vi "practiceImageAnalysis.vi"() -> ()   [LabVIEW 2016]
uses:
  <vilib>/regexp/Match Regular Expression.xnode
  <vilib>/Utility/file.llb/Write Delimited Spreadsheet (DBL).vi
  <vilib>/vision/Measure.llb/Straight Edge Process.ctl
  <vilib>/vision/Measure.llb/Straight Edge Options.ctl
  <vilib>/vision/Measure.llb/Edge Polarity.ctl
  <vilib>/vision/Measure.llb/Edge Options.ctl
panel:
  out "Coordinate array for image capture":dbl[][](array[numeric])
  in  "Coordinate file for image capture":path=path "E:/XYZstage+Camera_CollectedImages/12-16-2016/noStaveMount/toolingpinsCoordinates-captured.csv"
  out "Review":bool
  out "Search running?":bool
  in  "Options: Bottom Edge Search":T3={"Search Direction"=3, "Edge Options"={"Edge Polarity"=2, "Kernel Size"=9, "Width"=3, "Minimum Edge Strength"=17.0, "Interpolation Type"=enum."Bilinear Fixed", "Data Processing Method"=enum."Average"}, "Show Search Area"=TRUE, "Show Search Lines"=TRUE, "Show Edges Found"=TRUE, "Show Result"=TRUE, "Search Area Color"=65280, "Search Lines Color"=255, "Edge Locations Color"=16776960, "Result Color"=16711680, "Overlay Group Name"=""} {"Search Direction" items=["Left to Right", "Right to Left", "Top to Bottom", "Bottom to Top"]; "Edge Options"."Edge Polarity" items=["All Edges", "Rising Edges", "Falling Edges"]; "Edge Options"."Minimum Edge Strength" format="%.2f"; "Edge Options"."Width" step=2; "Edge Options"."Kernel Size" step=2}
  in  "Options: Top Edge Search":T3={"Search Direction"=2, "Edge Options"={"Edge Polarity"=0, "Kernel Size"=5, "Width"=3, "Minimum Edge Strength"=16.0, "Interpolation Type"=enum."Bilinear Fixed", "Data Processing Method"=enum."Average"}, "Show Search Area"=TRUE, "Show Search Lines"=TRUE, "Show Edges Found"=TRUE, "Show Result"=TRUE, "Search Area Color"=65280, "Search Lines Color"=255, "Edge Locations Color"=16776960, "Result Color"=16711680, "Overlay Group Name"=""} {"Search Direction" items=["Left to Right", "Right to Left", "Top to Bottom", "Bottom to Top"]; "Edge Options"."Edge Polarity" items=["All Edges", "Rising Edges", "Falling Edges"]; "Edge Options"."Minimum Edge Strength" format="%.2f"; "Edge Options"."Width" step=2; "Edge Options"."Kernel Size" step=2}
  in  "Fit Options":T4={"Number of Lines"=1, "Type"=enum."First Edge Rake", "Min. Score"=10.0, "Max. Score"=1000.0, "Orientation"=0.0, "Angle Range"=45.0, "Angle Tolerance"=1.0, "Step Size"=196, "Min. SNR (db)"=0.0, "Min. Points (%)"=25.0, "Hough Iterations"=5} {"Min. Points (%)" min=0.0 max=100.0; "Min. SNR (db)" min=0.0; "Max. Score" min=0.0 max=1024.0; "Min. Score" min=0.0 max=1024.0 step=1.0}
  in  "Stop and delete":bool
  out "Images Array":T6[](array[plugin-control])
  in  "error in":errorcluster
  out "error out":errorcluster
  out "Filenames Array":string[](array[string])
  in  "Naming Convention":string="*.png"
  in  "Images Directory":path=path "E:/XYZstage+Camera_CollectedImages/12-16-2016/noStaveMount/toolingpins_images"
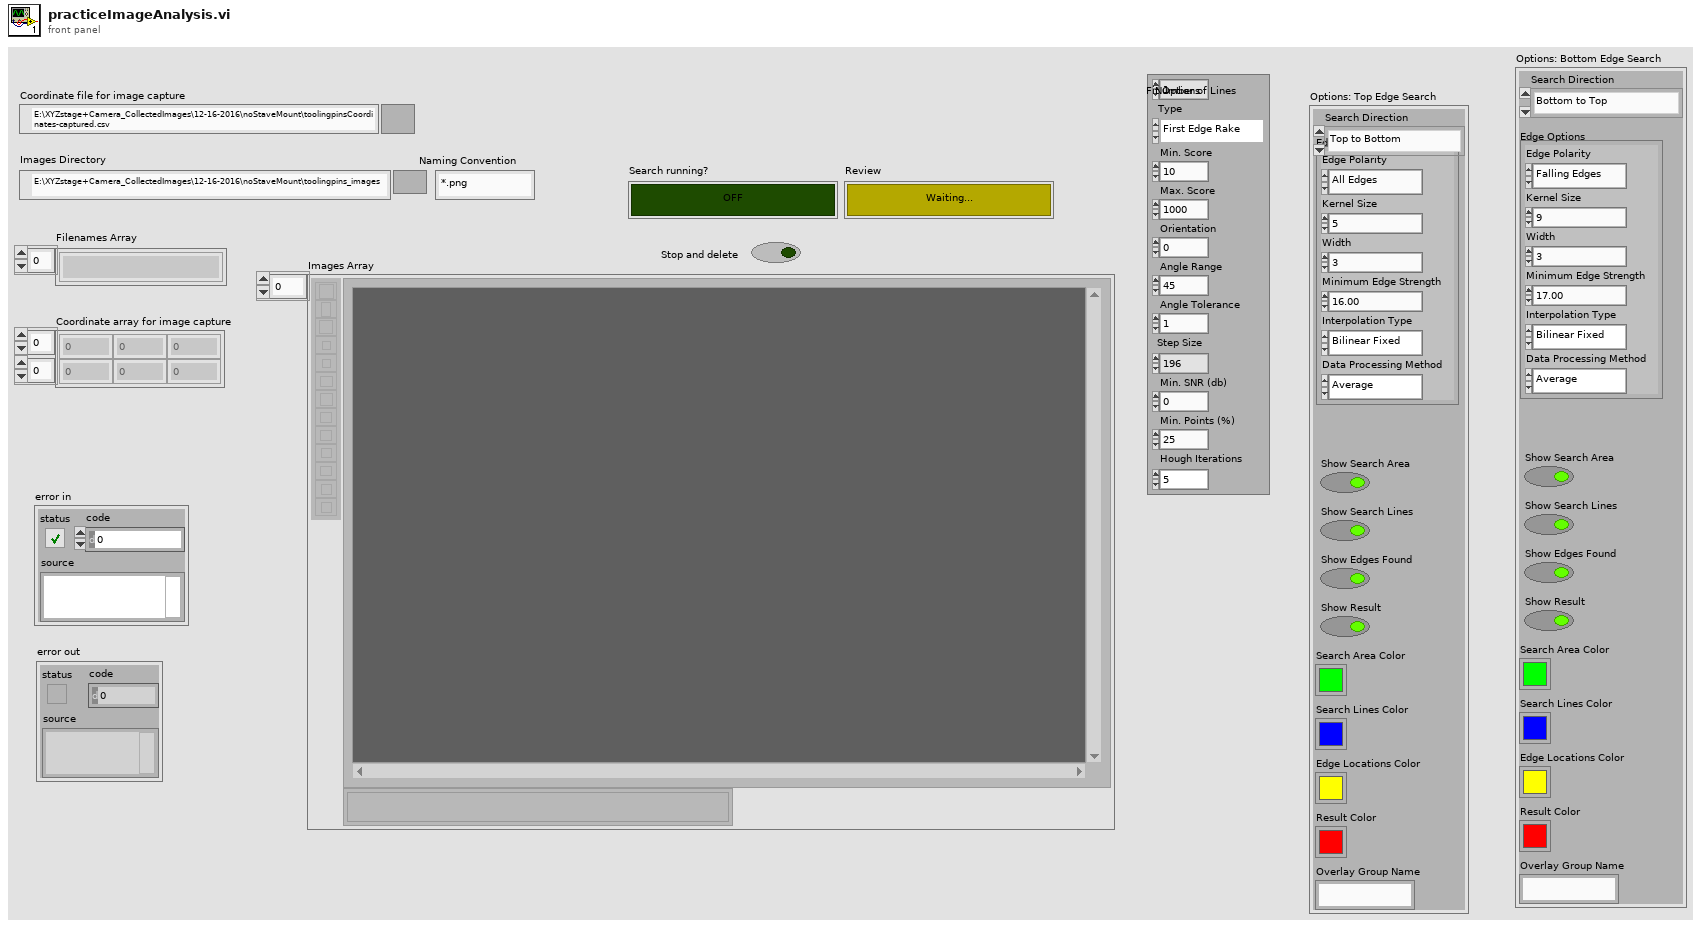
[diagram p1: front panel]
types:
  T1 = typedef "Edge Options.ctl" = cluster{"Edge Polarity":T2, "Kernel Size":u32, "Width":u32, "Minimum Edge Strength":sgl, "Interpolation Type":enum32{"Zero Order", "Bilinear", "Quadratic", "Cubic", "Bilinear Fixed"}, "Data Processing Method":enum32{"Average", "Median"}}
  T2 = typedef "Edge Polarity.ctl" = u32
  T3 = cluster{"Search Direction":u32, "Edge Options":T1, "Show Search Area":bool, "Show Search Lines":bool, "Show Edges Found":bool, "Show Result":bool, "Search Area Color":u32, "Search Lines Color":u32, "Edge Locations Color":u32, "Result Color":u32, "Overlay Group Name":string}
  T4 = typedef "Straight Edge Options.ctl" = cluster{"Number of Lines":i32, "Type":T5, "Min. Score":dbl, "Max. Score":dbl, "Orientation":dbl, "Angle Range":dbl, "Angle Tolerance":dbl, "Step Size":u32, "Min. SNR (db)":dbl, "Min. Points (%)":dbl, "Hough Iterations":i32}
  T5 = typedef "Straight Edge Process.ctl" = enum32{"First Edge Rake", "Best Edge Rake", "Hough Edge Rake", "First Edge Projection", "Best Edge Projection"}
  T6 = typedef "IMAQ Image.ctl" = refnum<image>
  T7 = enum16{"cm", "mm", "pixels [mm/pix]", "pixels [um/pix]"}
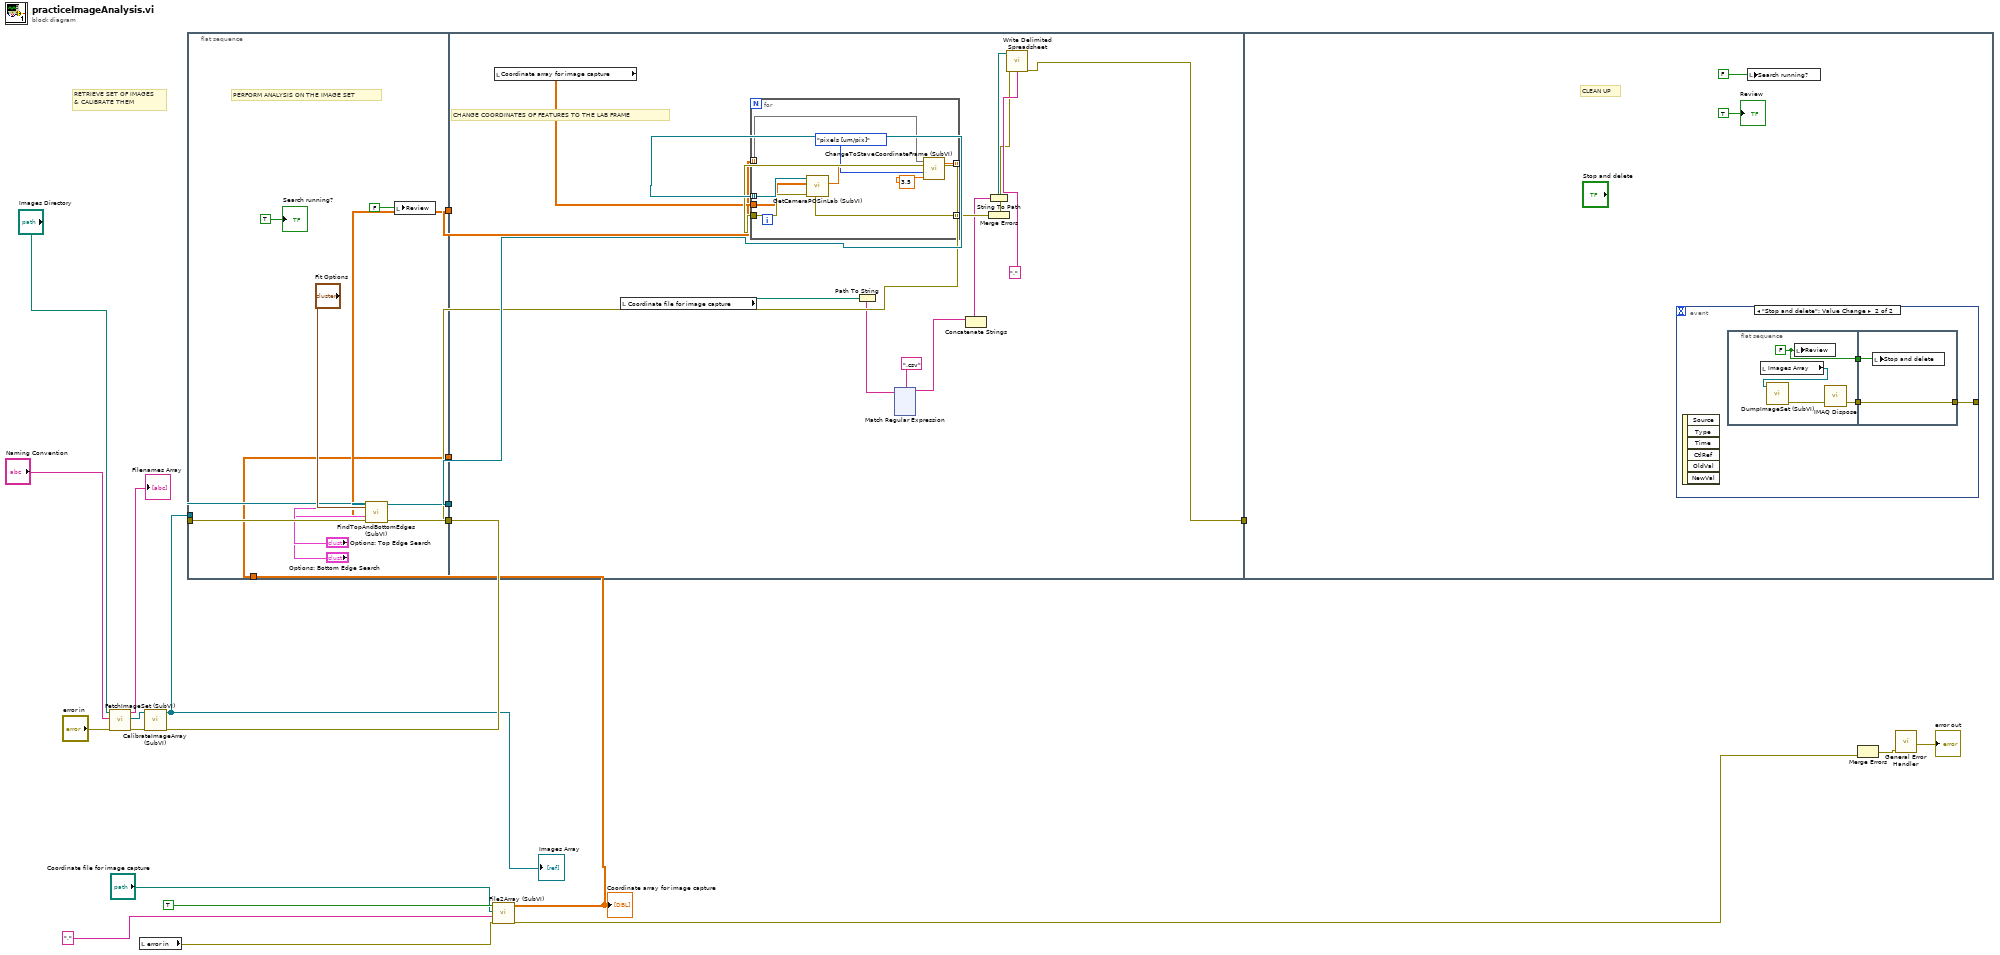
[diagram p0: block diagram]
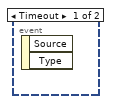
[diagram p2: hidden frame]
diagram:
  # "RETRIEVE SET OF IMAGES\n& CALIBRATE THEM"
  n1 = call "FetchImageSet (SubVI).vi"("error in (no error)"="error in", "Naming Convention"="Naming Convention", "Images Directory"="Images Directory") -> ("error out"=w17:errorcluster, "Image Array"=w18:T6[], "Filenames Array"=→"Filenames Array":string[])  [unwired: 6 in]
  n2 = local read "error in"() -> (w7:errorcluster)
  n3 = call "CalibrateImageArray (SubVI).vi"("error in (no error)"=w17, "Image Array"=w18) -> ("error out"=w14:errorcluster, "Calibrated Image Array"=w13:T6[])  [unwired: 7 in]
  "Images Array" <- w13
  n4 = flat-sequence {
    tunnel: w14 -> [w32]
    tunnel: w13 -> [w24]
    tunnel: [w31] -> w12
    tunnel: [w30] -> w11
    tunnel: [w23] -> w4
    tunnel: w2 -> [w22]
    tunnel: [w22] -> w1
    tunnel: w12 -> [w45]
    tunnel: w11 -> [w46]
    tunnel: w4 -> [w43]
    tunnel: [w33] -> w3
    tunnel: w1 -> [_]
    tunnel: w3 -> [_]
    frame #0 {
      # "PERFORM ANALYSIS ON THE IMAGE SET"
      n5 = call "FindTopAndBottomEdges (SubVI).vi"("Calibrated Image Array"=w24, "Fit Options"="Fit Options", "Options: Top Edge Search"="Options: Top Edge Search", "Options: Bottom Edge Search"="Options: Bottom Edge Search", "error in (no error)"=w32) -> ("Analyzed Image Array"=w30:T6[], "Array of Edge Endpoint Arrays"=w23:sgl[][][], "error out"=w31:errorcluster)  [unwired: 6 in, 2 out]
      n6 = local write "Review"(FALSE ("Review")) -> ()
      "Search running?" <- TRUE ("Search running?")
    }
    frame #1 {
      # "CHANGE COORDINATES OF FEATURES TO THE LAB FRAME"
      n7 = local read "Coordinate array for image capture"() -> (w44:dbl[][])
      n8 = local read "Coordinate file for image capture"() -> (w41:path)
      n9 = for {
        tunnel: w46 -> [w169] mode=indexing
        tunnel: w45 -> [w168]
        tunnel: w44 -> [w167]
        tunnel: w43 -> [w165] mode=indexing
        tunnel: [w162] -> w42 mode=indexing
        tunnel: [w161] -> _ mode=indexing
        n10 = call "GetCameraPOSinLab (SubVI).vi"("error in (no error)"=w168, "Loaded array"=w167, "Refnum in"=w169) -> ("error out"=w162:errorcluster, "Image coordinates in lab frame"=w166:dbl[])  [unwired: 6 in, 1 out]
        n11 = call "ChangeToStaveCoordinateFrame (SubVI).vi"("Array (image frame, specified units)"=w165, "Image Origin in XYZ Stage Coords [mm]"=w166, "Units"=T7."pixels [um/pix]", "Pixel resolution"=3.5) -> ("Array (stage frame, mm)"=w161:dbl[][])  [unwired: 2 in]
      }
      n12 = Path To String(path=w41) -> (string=w39:string)
      n13 = xnode "Match Regular Expression"("input string"=w39, "regular expression"=".csv") -> ("before match"=w38:string)  [unwired: 4 in, 4 out]
      n14 = Concatenate Strings(w38) -> (w37:string)  [unwired: 1 in]
      n15 = String To Path(string=w37) -> (path=w35:path)
      n16 = Merge Errors(w42) -> (w34:errorcluster)
      n17 = call-poly <vilib>:"Write Delimited Spreadsheet.vi"("file path (dialog if empty)"=w35, "error in (no error)"=w34, "delimiter (\\t)"="," ("delimiter (\\t)")) -> ("error out"=w33:errorcluster)  [unwired: 11 in, 1 out]
    }
    frame #2 {
      # "CLEAN UP"
      n18 = event shown="[1] \"Stop and delete\": Value Change" {
        selector: _ -> [_ _]
        dyn-events: _ -> [_ _]
        timeout: _ -> [_ _]
        tunnel: [_ w172] -> _
        event Timeout {
          n19 = event-data() -> ()  [unwired: 1 in, 2 out]
        }
        event "Stop and delete": Value Change {
          n20 = event-data() -> ()  [unwired: 1 in, 6 out]
          n21 = flat-sequence {
            tunnel: [w178] -> w174
            tunnel: [w176] -> w173
            tunnel: w174 -> [w180]
            tunnel: w173 -> [w179]
            tunnel: [w179] -> w172
            frame #0 {
              w178 = FALSE ("Review")
              n22 = local read "Images Array"() -> (w175:T6[])
              n23 = call "DumpImageSet (SubVI).vi"("Calibrated Image Array"=w175) -> ("error out"=w177:errorcluster)  [unwired: 7 in]
              n24 = local write "Review"(w178) -> ()
              n25 = call "IMAQ Dispose"("error in (no error)"=w177) -> ("error out"=w176:errorcluster)  [unwired: 5 in]
            }
            frame #1 {
              n26 = local write "Stop and delete"(w180) -> ()
            }
          }
        }
      }
      n27 = local write "Search running?"(FALSE ("Search running?")) -> ()
      "Review" <- TRUE ("Review")
    }
  }
  n28 = call "File2Array (SubVI).vi"("error in (no error) in"=w7, "File delimiter"=",", "Source array file"="Coordinate file for image capture", "Load array from file?"=TRUE) -> ("error in (no error) out"=w6:errorcluster, "Loaded array"=w2:dbl[][])  [unwired: 6 in]
  "Coordinate array for image capture" <- w2
  n29 = Merge Errors(w6) -> (w5:errorcluster)  [unwired: 1 in]
  n30 = call <vilib>:"General Error Handler.vi"("error in (no error)"=w5) -> ("error out"=→"error out":errorcluster)  [unwired: 10 in, 4 out]
